vi "DDC.vi"(7 "reset":bool, 9 "DDC params":T1 {"output sample rate" format="%.48g"; "frequency shift" format="%#.48g"}, 10 ">> rx start trigger >>":bool, 11 "IQ":T2) -> (2 "output valid":bool, 3 "data out":T2)   [LabVIEW 2021]
uses:
  <instrlib>/_niInstr/DSP/v1/Shared/Public/IQ Data.ctl
  <instrlib>/_niInstr/DSP/v1/FPGA/Public/Sub VIs/Frequency Shift/Frequency Shift - 1 spc.vi
  <instrlib>/_niInstr/DSP/v1/FPGA/Public/Sub VIs/Fractional Decimator/Fractional Decimator - 1 spc - 2x oc.vi
  <instrlib>/_niInstr/DSP/v1/Xnodes/Public/Decimator/niInstr DSP v1 Decimator FPGA.xnode
  <instrlib>/_niInstr/Basic Elements/v1/FPGA/niInstr Basic Elements v1 FPGA.lvlib
  <instrlib>/_niInstr/DSP/v1/FPGA/niInstr DSP v1 FPGA.lvlib
  <instrlib>/_niInstr/DSP/v1/Shared/niInstr DSP v1 Shared.lvlib
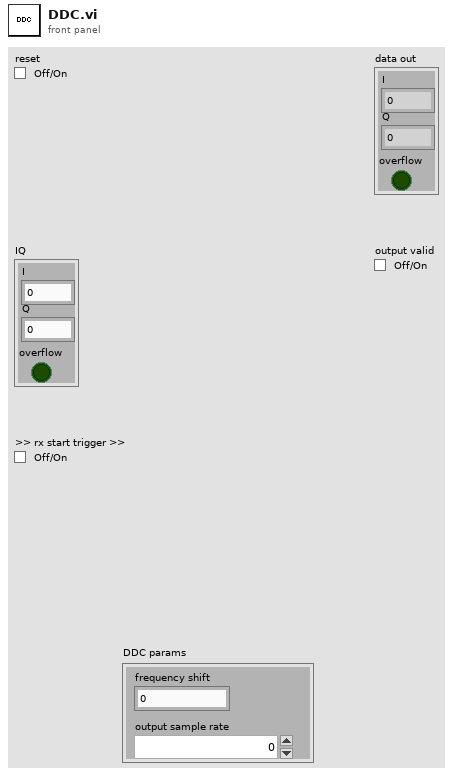
[diagram p1: front panel]
types:
  T1 = cluster{"frequency shift":fxp<+/-,48,0>, "output sample rate":fxp<+,48,1>}
  T2 = typedef "niInstr DSP v1 Shared.lvlib/IQ Data.ctl" = cluster{"I":fxp<+/-,18,1>, "Q":fxp<+/-,18,1>, "overflow":bool}
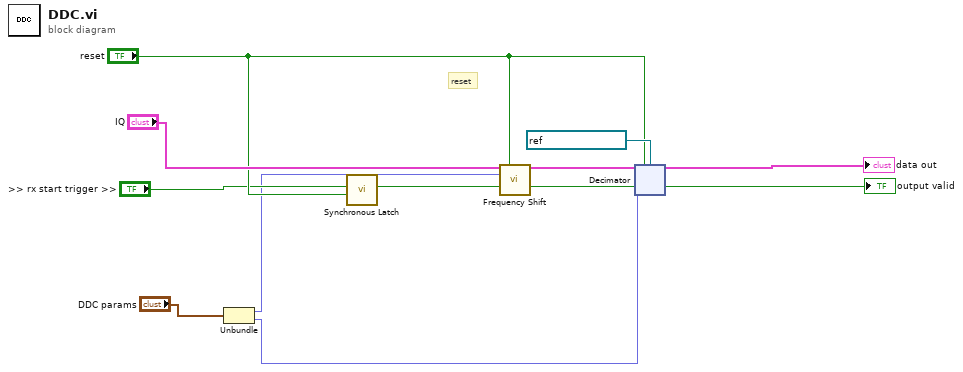
[diagram p0: block diagram]
diagram:
  # "reset"
  n1 = Unbundle("DDC params") -> ("frequency shift"=w2:fxp<+/-,48,0>, "output sample rate"=w1:fxp<+,48,1>)
  n2 = call <instrlib>:"Synchronous Latch.vi"("clear"="reset", "set"=">> rx start trigger >>") -> ("out"=w4:bool)  [unwired: 9 in]
  n3 = call-poly <instrlib>:"Frequency Shift.vi"("data in"="IQ", "reset"="reset", "frequency shift"=w2, "input valid"=w4) -> ("data out"=w7:T2, "output valid"=w8:bool)  [unwired: 8 in, 2 out]
  n4 = xnode "Decimator"("data in"=w7, "reset"="reset", "input valid"=w8, "output sample rate"=w1, "clock x2"=refnum<k21> "Data Clock x2" ("oversample clock")) -> ("data out"=→"data out":T2, "output valid"=→"output valid":bool)  [unwired: 1 in, 1 out]
